vi "Get Displayed Sequence.vi"(8 "error in (no error)":errorcluster, 11 "SequenceViewPanel in":refnum<class "SequenceViewPanel.lvclass">) -> (0 "error out":errorcluster, 2 "Sequence":string, 3 "SequenceViewPanel out":refnum<class "SequenceViewPanel.lvclass">)   [LabVIEW 2020, in "TSnax UI.lvlib" / "SequenceViewPanel.lvclass"]
uses:
  SequenceViewPanel.lvclass
  SequenceViewPanel.lvclass/SequenceViewPanel.ctl
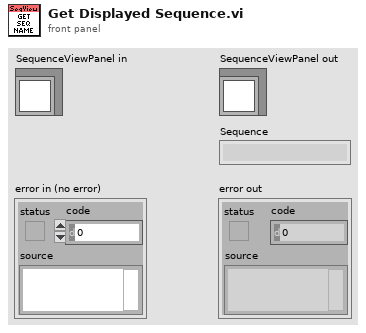
[diagram p1: front panel]
types:
  T1 = typedef "TSnax UI.lvlib/SequenceViewPanel.lvclass/Ref Data.ctl" = cluster{"Insert Index":i32, "SequenceFile":refnum<class "SequenceFile.lvclass">, "Sequence":string}
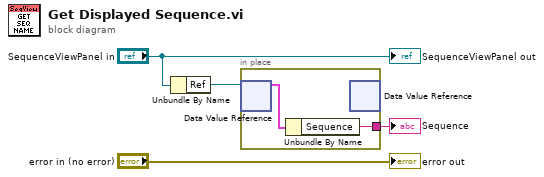
[diagram p0: block diagram]
diagram:
  n1 = Unbundle By Name("SequenceViewPanel in") -> ("Ref"=w3:refnum<data-value>)
  n2 = in-place {
    in-place-border: [w5] -> w1
    n3 = in-place-dvr #1(w3) -> (w6:T1)  [unwired: 1 out]
    n4 = Unbundle By Name(w6) -> ("Sequence"=w5:string)
    n5 = in-place-dvr #1() -> ()  [unwired: 1 in, 2 out]
  }
  "Sequence" <- w1
  "error out" <- "error in (no error)"
  "SequenceViewPanel out" <- "SequenceViewPanel in"
